vi "test_Remove Waveform Output Channels.vi"(8 "error in (no error)":errorcluster, 11 "TestCase in":refnum<class "FPGA Addon Adding Channel Items Unit Tests.lvclass">=refnum) -> (0 "error out":errorcluster, 3 "TestCase out":refnum<class "FPGA Addon Adding Channel Items Unit Tests.lvclass">)   [LabVIEW 2019, in "FPGA Addon Adding Channel Items Unit Tests.lvclass"]
uses:
  FPGA Addon Adding Channel Items Unit Tests.lvclass
  <vilib>/addons/_JKI Toolkits/VI Tester/TestCase.llb/TestCase.lvclass
  <vilib>/NI VeriStand/Custom Device Tools/Custom Device Utility Library/Custom Device Utility Library.lvlib
  Addon/Addon Shared/SubVIs/Constants.vi
  Addon/Addon Shared/FPGA Addon Shared.lvlib
  <vilib>/NI/NI VeriStand Advanced SysDef API/SysDef API/Advanced System Definition.lvlib
  <vilib>/NI VeriStand/Custom Device Tools/Custom Device Utility Library/NI VeriStand - Search for Item by GUID.vi
  Addon/Addon System Explorer/FPGA Addon System Explorer.lvlib
  <vilib>/NI VeriStand/Custom Device API/Custom Device Item Ref.ctl
  <vilib>/NI VeriStand/Custom Device API/Custom Device API.lvlib
  Addon/Addon System Explorer/Types/SE UI Cluster.ctl
  <vilib>/NI/NI VeriStand Advanced SysDef API/_SubVIs/SysDef.Search.GUIDs.vi
panel:
  out "GUIDs":string[](array[string])
  in  "remove":bool
  in  "add":bool
  out "Names":string[](array[string])
  in  "Available Registers":i32[](listbox)
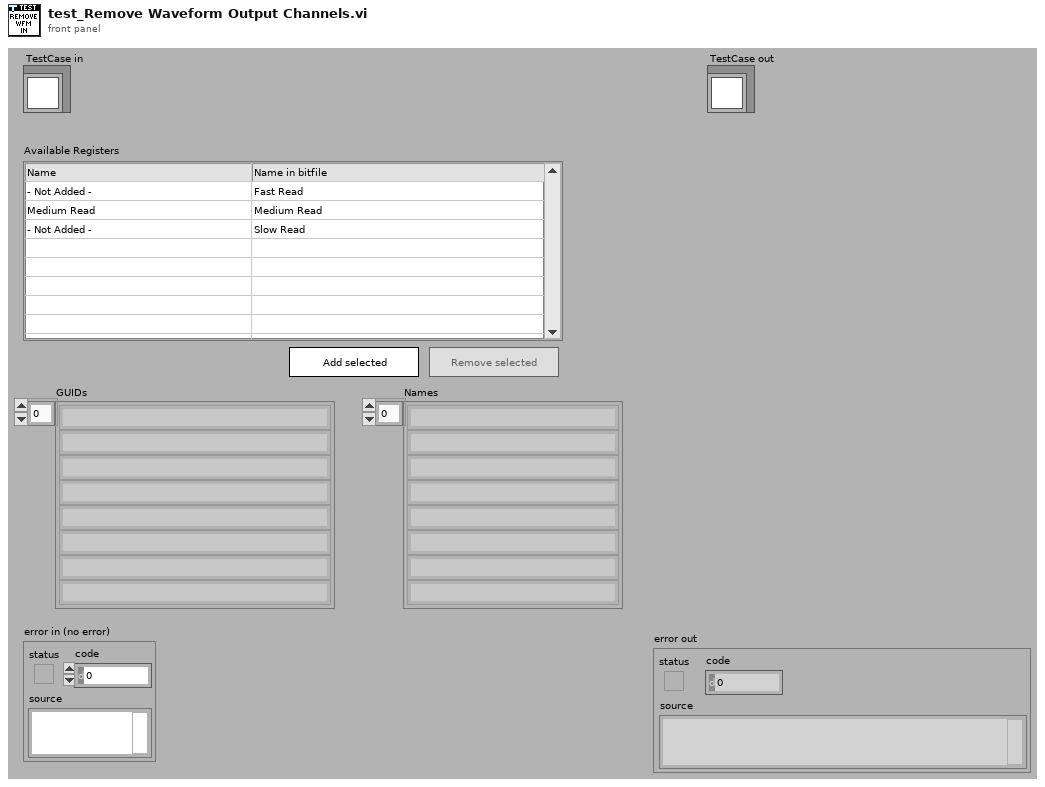
[diagram p1: front panel]
types:
  T1 = typedef "FPGA Addon System Explorer.lvlib/SE UI Cluster.ctl" = cluster{"Node Ptr":T2, "Add":refnum<vi>, "Remove":refnum<vi>, "Registers ListBox":refnum<vi>}
  T2 = typedef "Custom Device API.lvlib/Custom Device Item Ref.ctl" = u64
  T3 = typedef "Advanced System Definition.lvlib/TreeItem.Info.ctl" = cluster{"Name":string, "Description":string, "GUID":string, "Is Channel":bool, "Channel":T4, "Is Waveform":bool, "Waveform":T6}
  T4 = typedef "Custom Device API.lvlib/Custom Device Channel.ctl" = cluster{"Type":T5, "Units":string, "Default Value":dbl, "Faultable":bool, "Scalable":bool}
  T5 = typedef "Custom Device API.lvlib/Custom Device Channel Type.ctl" = enum16{"Input", "Output"}
  T6 = typedef "Custom Device API.lvlib/Custom Device Waveform.ctl" = cluster{"Data Type":T7, "Units":string}
  T7 = typedef "Custom Device API.lvlib/Custom Device Waveform DataType.ctl" = enum16{"Double", "Complex Double"}
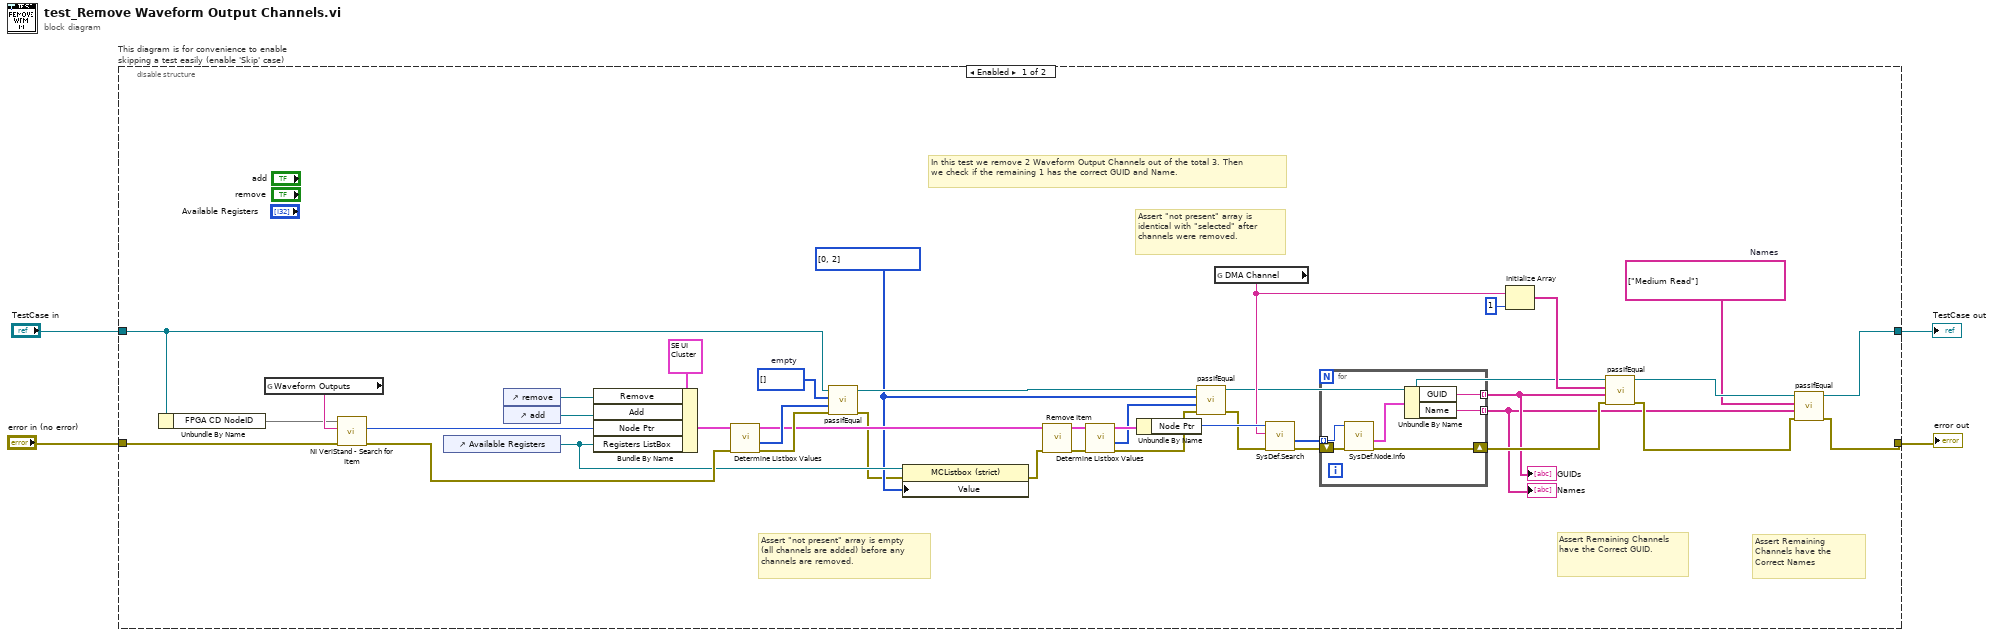
[diagram p0: block diagram]
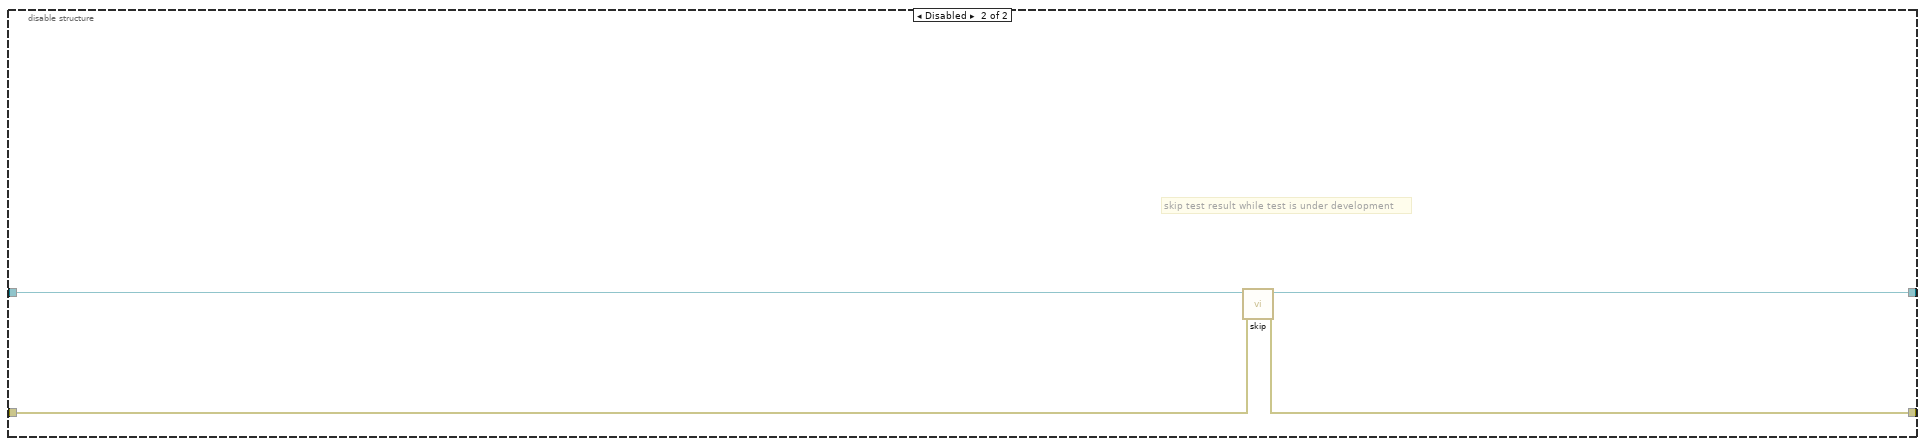
[diagram p2: hidden frame]
diagram:
  n1 = disable-structure "This diagram is for convenience to enable skipping a test easily (enable 'Skip' case)" shown="Enabled" {
    disable-tunnel: "TestCase in" -> [w24 w54]
    disable-tunnel: [w34 w52] -> w1
    disable-tunnel: [w33 w53] -> w3
    disable-tunnel: "error in (no error)" -> [w32 w51]
    frame Enabled {
      w25 = i32[] []  # empty
      w35 = string[] ["Medium Read"]  # Names
      w11 = i32[] [0, 2] ("selected")
      # "Assert \"not present\" array is empty (all channels are added) before any channels are removed."
      # "Assert \"not present\" array is identical with \"selected\" after channels were removed."
      # "In this test we remove 2 Waveform Output Channels out of the total 3. Then we check if the remaining 1 has the correct GUID and Name."
      # "Assert Remaining Channels have the Correct Names"
      # "Assert Remaining Channels have the Correct GUID."
      n2 = Unbundle By Name(w24) -> ("FPGA CD NodeID"=w31)
      n3 = global read "Constants.vi" "Waveform Outputs"() -> (w44:string)
      n4 = call-poly <vilib>:"NI VeriStand - Search for Item.vi"("error in"=w32, "Item GUID"=w44, "Section Ref in"=w31) -> ("error out"=w16:errorcluster, "Item Ref"=w19:T2)  [unwired: 5 in, 2 out]
      n5 = control-ref of="Available Registers"() -> (w12:refnum<vi>)
      n6 = control-ref of="remove"() -> (w18:refnum<vi>)
      n7 = control-ref of="add"() -> (w17:refnum<vi>)
      n8 = Bundle By Name(cluster=T1 {"Node Ptr"=18446744073709551615, "Add"=refnum, "Remove"=refnum, "Registers ListBox"=refnum} ("SE UI cluster in"), "Remove"=w18, "Add"=w17, "Node Ptr"=w19, "Registers ListBox"=w12) -> (w15:T1)
      n9 = call "Determine Listbox Values.vi"("error in (no error)"=w16, "SE UI cluster in"=w15) -> ("error out"=w21:errorcluster, "Not imported item Indexes"=w22:i32[], "SE UI cluster out"=w14:T1)  [unwired: 6 in, 1 out]
      n10 = call-dynamic "passIfEqual.vi"("error in (no error)"=w21, "y"=w22, "x"=w25, "TestCase in"=w24) -> ("error out"=w5:errorcluster, "TestCase out"=w23:refnum<class "FPGA Addon Adding Channel Items Unit Tests.lvclass">)  [unwired: 6 in]
      n11 = property class="MCListbox (strict)"(reference=w12, error in=w5, "Value"=w11) -> (error out=w13:errorcluster)  [unwired: 1 out]
      n12 = call "Remove Item.vi"("error in (no error)"=w13, "SE UI cluster in"=w14) -> ("error out"=w9:errorcluster, "SE UI cluster out"=w10:T1)  [unwired: 7 in, 1 out]
      n13 = call "Determine Listbox Values.vi"("error in (no error)"=w9, "SE UI cluster in"=w10) -> ("error out"=w7:errorcluster, "Not imported item Indexes"=w6:i32[], "SE UI cluster out"=w8:T1)  [unwired: 6 in, 1 out]
      n14 = Unbundle By Name(w8) -> ("Node Ptr"=w42:T2)
      n15 = call-dynamic "passIfEqual.vi"("error in (no error)"=w7, "y"=w6, "x"=w11, "TestCase in"=w23) -> ("error out"=w27:errorcluster, "TestCase out"=w26:refnum<class "FPGA Addon Adding Channel Items Unit Tests.lvclass">)  [unwired: 6 in]
      n16 = global read "Constants.vi" "DMA Channel"() -> (w29:string)
      n17 = call-poly <vilib>:"SysDef.Search.vi"("error in (no error)"=w27, "GUID"=w29, "nodeID"=w42) -> ("error out"=w43:errorcluster, "Values Out"=w41:u64[])  [unwired: 5 in, 2 out]
      n18 = for {
        tunnel: w41 -> [w47] mode=indexing
        tunnel: [w45] -> w36 mode=indexing
        tunnel: [w46] -> w38 mode=indexing
        shift-right: [w49] -> w39
        shift-left: w43 -> [w50]
        n19 = call <vilib>:"SysDef.Node.Info.vi"("error in (no error)"=w50, "nodeID"=w47) -> ("error out"=w49:errorcluster, "Item Info"=w48:T3)  [unwired: 6 in, 2 out]
        n20 = Unbundle By Name(w48) -> ("GUID"=w46:string, "Name"=w45:string)
      }
      "Names" <- w36
      "GUIDs" <- w38
      n21 = Initialize Array(w29, 1 ("dimension size")) -> (w30:string[])
      n22 = call-dynamic "passIfEqual.vi"("error in (no error)"=w39, "y"=w38, "x"=w30, "TestCase in"=w26) -> ("error out"=w40:errorcluster, "TestCase out"=w37:refnum<class "FPGA Addon Adding Channel Items Unit Tests.lvclass">)  [unwired: 6 in]
      n23 = call-dynamic "passIfEqual.vi"("error in (no error)"=w40, "y"=w36, "x"=w35, "TestCase in"=w37) -> ("error out"=w33:errorcluster, "TestCase out"=w34:refnum<class "FPGA Addon Adding Channel Items Unit Tests.lvclass">)  [unwired: 6 in]
    }
    frame Disabled {
      # "skip test result while test is under development"
      n24 = call <vilib>:"skip.vi"("error in (no error)"=w51, "TestCase in"=w54) -> ("error out"=w53:errorcluster, "TestCase out"=w52:refnum<class "TestCase.lvclass">)  [unwired: 8 in]
    }
  }
  "error out" <- w3
  "TestCase out" <- w1
